vi "Set Mapping Targets.vi"(8 "error in (no error)":errorcluster, 10 "Mapping Targets":refnum<class "Sub Object.lvclass">[](array[class]), 11 "PDO Mapping in":refnum<class "PDO Mapping.lvclass">) -> (0 "error out":errorcluster, 3 "PDO Mapping out":refnum<class "PDO Mapping.lvclass">)   [LabVIEW 2020, in "CANopen.lvlib" / "PDO Mapping.lvclass"]
uses:
  PDO Mapping.lvclass
  Sub Object/Sub Object.lvclass
  PDO Mapping.lvclass/PDO Mapping.ctl
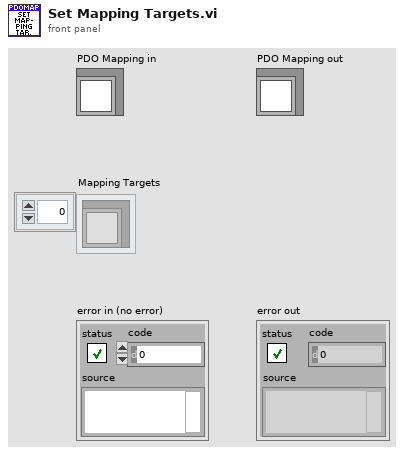
[diagram p1: front panel]
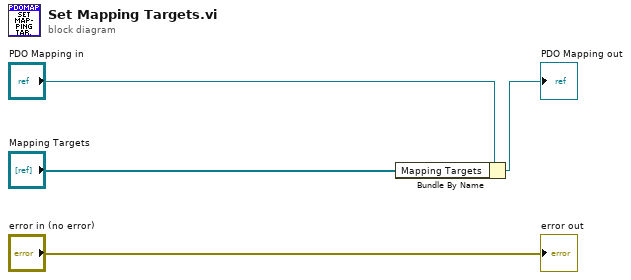
[diagram p0: block diagram]
diagram:
  n1 = Bundle By Name(cluster="PDO Mapping in", "Mapping Targets"="Mapping Targets") -> (→"PDO Mapping out":refnum<class "PDO Mapping.lvclass">)
  "error out" <- "error in (no error)"
